vi "Get Data Queue.vi"(8 "error in (no error)":errorcluster, 10 "Target Name":string, 11 "Task Base in":refnum<class "Task Base.lvclass">) -> (0 "error out":errorcluster, 2 "Data Queue":refnum<queue>, 3 "Task Base out":refnum<class "Task Base.lvclass">)   [LabVIEW 2023, in "HAL GOOP4.lvlib" / "Task Base.lvclass"]
uses:
  Task Base.lvclass
  Task Base.lvclass/Task Base.ctl
  <vilib>/Utility/error.llb/Error Cluster From Error Code.vi
  <vilib>/ErrorRing/Error Ring.xnode
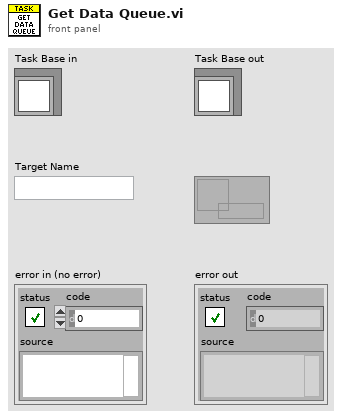
[diagram p1: front panel]
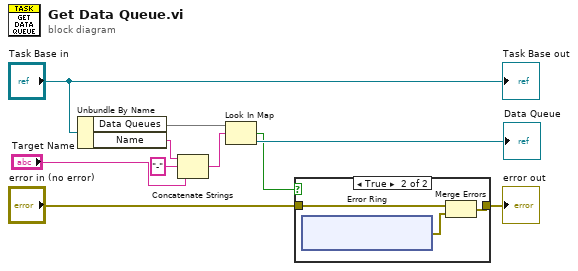
[diagram p0: block diagram]
diagram:
  n1 = Unbundle By Name("Task Base in") -> ("Data Queues"=w8:map{string, refnum<queue>}, "Name"=w4:string)
  n2 = Concatenate Strings(w4, "-" ("string"), "Target Name") -> (w3:string)
  n3 = Look In Map(map=w8, key=w3) -> (key not found?=w5:bool, value=→"Data Queue":refnum<queue>)  [unwired: 1 in]
  n4 = case shown="True" w5 {
    tunnel: "error in (no error)" -> [w11 w14]
    tunnel: [w11 w13] -> w6
    frame False {
    }
    frame True {
      n5 = xnode "Error Ring"() -> ("error out"=w12:errorcluster)
      n6 = Merge Errors(w14, w12) -> (w13:errorcluster)
    }
  }
  "error out" <- w6
  "Task Base out" <- "Task Base in"
